vi "Read D.vi"(8 "error in (no error)":errorcluster, 11 "Update PID CMD in":refnum<class "Update PID CMD.lvclass">) -> (0 "error out":errorcluster, 2 "D":sgl, 3 "Update PID CMD out":refnum<class "Update PID CMD.lvclass">)   [LabVIEW 2014, in "Humidifier Lib.lvlib" / "Update PID CMD.lvclass"]
uses:
  Update PID CMD.lvclass
  Update PID CMD.lvclass/Update PID CMD.ctl
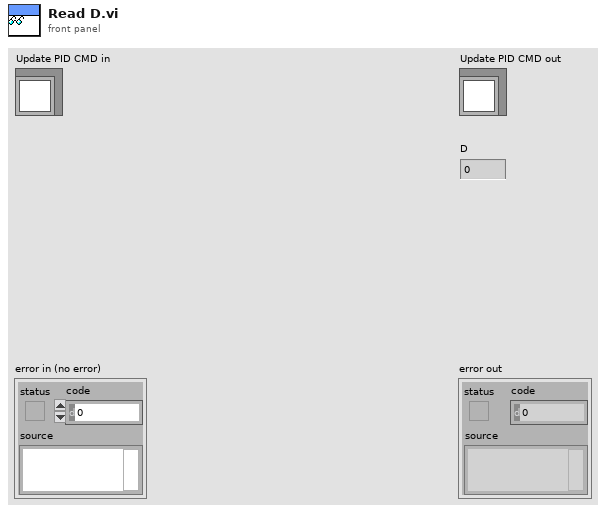
[diagram p1: front panel]
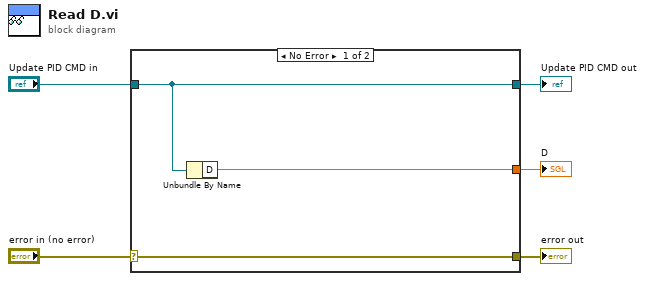
[diagram p0: block diagram]
diagram:
  n1 = case shown="No Error" "error in (no error)" {
    selector: "error in (no error)" -> [w8 w9]
    tunnel: [w8 w9] -> w4
    tunnel: [w7 w10] -> w2
    tunnel: "Update PID CMD in" -> [w7 w10]
    tunnel: [w6 _] -> w1
    frame No Error {
      n2 = Unbundle By Name(w7) -> ("D"=w6:sgl)
    }
    frame Error {
    }
  }
  "error out" <- w4
  "Update PID CMD out" <- w2
  "D" <- w1
